vi "CheckForInbit.vi"(1 "Action":T1={"Macro Instructions"=[{"Duration (s)"=1.0, "Steps"=1, "Changes"=[TRUE, FALSE], "Triggers"=[FALSE, FALSE, FALSE, FALSE, FALSE, FALSE, FALSE, FALSE, FALSE, FALSE, FALSE, FALSE, TRUE, FALSE, FALSE, FALSE, FALSE, FALSE, FALSE, FALSE, FALSE, FALSE, FALSE, FALSE, FALSE, FALSE, FALSE, FALSE, FALSE, FALSE, FALSE, FALSE, FALSE, FALSE, FALSE, FALSE, FALSE, FALSE], "RAW cmds 2D"=[[0, 0, 0, 0, 0, 0, 0, 0], [0, 0, 0, 0, 0, 0, 0, 0]]}], "Slow AO Array"=[{"ao line"="ao0", "Duration, Gain, NewVal"=[0.0, 0.0]}, {"ao line"="ao1", "Duration, Gain, NewVal"=[0.0, 0.0]}, {"ao line"="ao2", "Duration, Gain, NewVal"=[0.0, 0.0]}, {"ao line"="0.000000E+0", "Duration, Gain, NewVal"=[0.0]}], "Duration (s)"=1.0, "Toggle"=FALSE} {"Slow AO Array"."Duration, Gain, NewVal" format="%#_3g"}) -> (0 "Inbit #":i32)   [LabVIEW 2018]
uses:
  ActionCluster.ctl
  Instructions_RT.ctl
  ParameterSubCluster.ctl
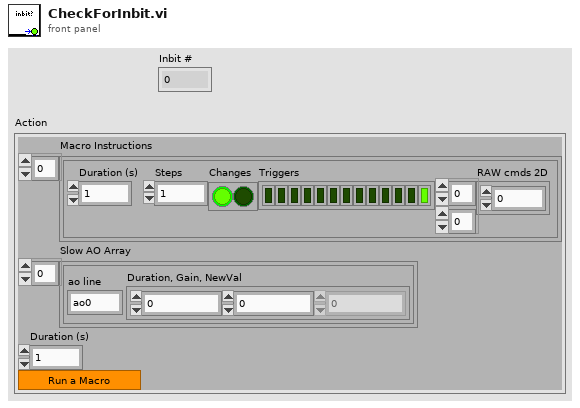
[diagram p1: front panel]
types:
  T1 = typedef "ActionCluster.ctl" = cluster{"Macro Instructions":T2, "Slow AO Array":T3, "Duration (s)":dbl, "Toggle":bool}
  T2 = typedef "Instructions_RT.ctl" = cluster{"Duration (s)":dbl, "Steps":i32, "Changes":bool[], "Triggers":bool[], "RAW cmds 2D":i16[][]}[]
  T3 = typedef "ParameterSubCluster.ctl" = cluster{"ao line":string, "Duration, Gain, NewVal":dbl[]}[]
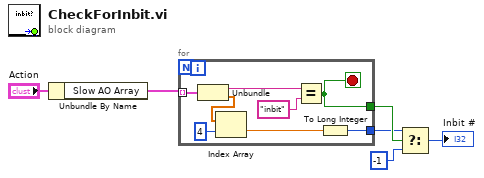
[diagram p0: block diagram]
diagram:
  n1 = Unbundle By Name("Action") -> ("Slow AO Array"=w5:T3)
  n2 = for {
    tunnel: w5 -> [w14] mode=indexing
    tunnel: [w12] -> w4
    tunnel: [w7] -> w3
    stop <- w12 stop-if-true
    n3 = Unbundle(w14) -> ("ao line"=w11:string, "Duration, Gain, NewVal"=w10:dbl[])
    n4 = Index Array(array=w10, index=4) -> (element=w8:dbl)
    n5 = Equal?(x=w11, y="inbit") -> (x = y?=w12:bool)
    n6 = To Long Integer(number=w8) -> (32bit integer=w7:i32)
  }
  n7 = Select(t=w3, s=w4, f=-1) -> (s? t:f=→"Inbit #":i32)
